vi "Configure Multitone Export.vi"(5 "Dither (0: dgNoDither)":i32(ring) items=["dgNoDither", "dgTriangular", "dgRectangular"], 6 "Number Of Bits (0)":i32, 7 "Mode (0: mtArbFile)":i32(ring) items=["mtArbFile", "mtWavFile"], 8 "error in (no error)":errorcluster, 9 "File Name (\"\")":string="\"\"", 10 "Channel (0: chA)":i32(ring) items=["chA", "chB"], 11 "VISA resource name":refnum<visa-resource-name>) -> (0 "error out":errorcluster, 3 "VISA resource name out":refnum<visa-resource-name>)   [LabVIEW 2014, in "Stanford Research SR1.lvlib"]
doc: "Exports the multitone waveformto either an arbitrary waveformor a .WAVfile with\nthe specified filename, bit resolution and dither options.\n\n<b>Note</b>: This Vi may not be supported by certain models of the SR1."
uses:
  Stanford Research SR1.lvlib
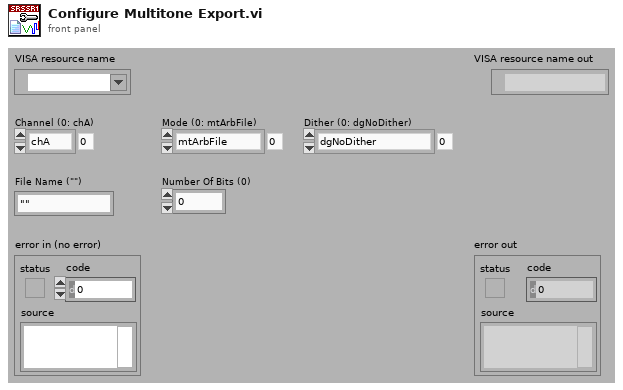
[diagram p1: front panel]
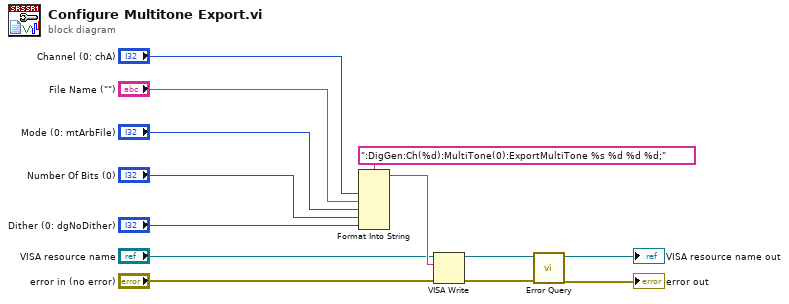
[diagram p0: block diagram]
diagram:
  n1 = Format Into String(format string=":DigGen:Ch(%d):MultiTone(0):ExportMultiTone %s %d %d %d;", "Channel (0: chA)", "File Name (\"\")", "Mode (0: mtArbFile)", "Number Of Bits (0)", "Dither (0: dgNoDither)") -> (resulting string=w12:string)  [unwired: 2 in, 1 out]
  n2 = VISA Write(VISA resource name="VISA resource name", write buffer=w12, error in (no error)="error in (no error)") -> (VISA resource name out=w9:refnum<visa-resource-name>, error out=w8:errorcluster)  [unwired: 1 out]
  n3 = call "Error Query.vi"("error in (no error)"=w8, "VISA resource name"=w9) -> ("error out"=→"error out":errorcluster, "VISA resource name out"=→"VISA resource name out":refnum<visa-resource-name>)  [unwired: 6 in, 2 out]
